vi "PAM Parse Other Data.vi"(1 "Header":string) -> (15 "Synchronization":T1, 16 "Magnetometer":T2, 17 "Acceleromter":T2)   [LabVIEW 2020]
panel:
  out "Sync Status":string
  out "System Time Status":string
  out "error out":errorcluster
  in  "error in (no error)":errorcluster
  out "Sync Offset":u32
  out "PPS Count":u32
  out "PPS Count":string
  out "Sync Offset":string
  out "Instrument Time":string
  out "Instrument Date":string
  out "Mag Z":i16
  out "Mag Y":i16
  out "Mag X":i16
  out "Accel Z":i16
  out "Accel Y":i16
  out "Accel X":i16
  out "Heading":string
  out "Battery":string
  out "Time":string
  out "Trigger Status":string
  out "Temp, Humidity":string
  out "Other Data Header":string
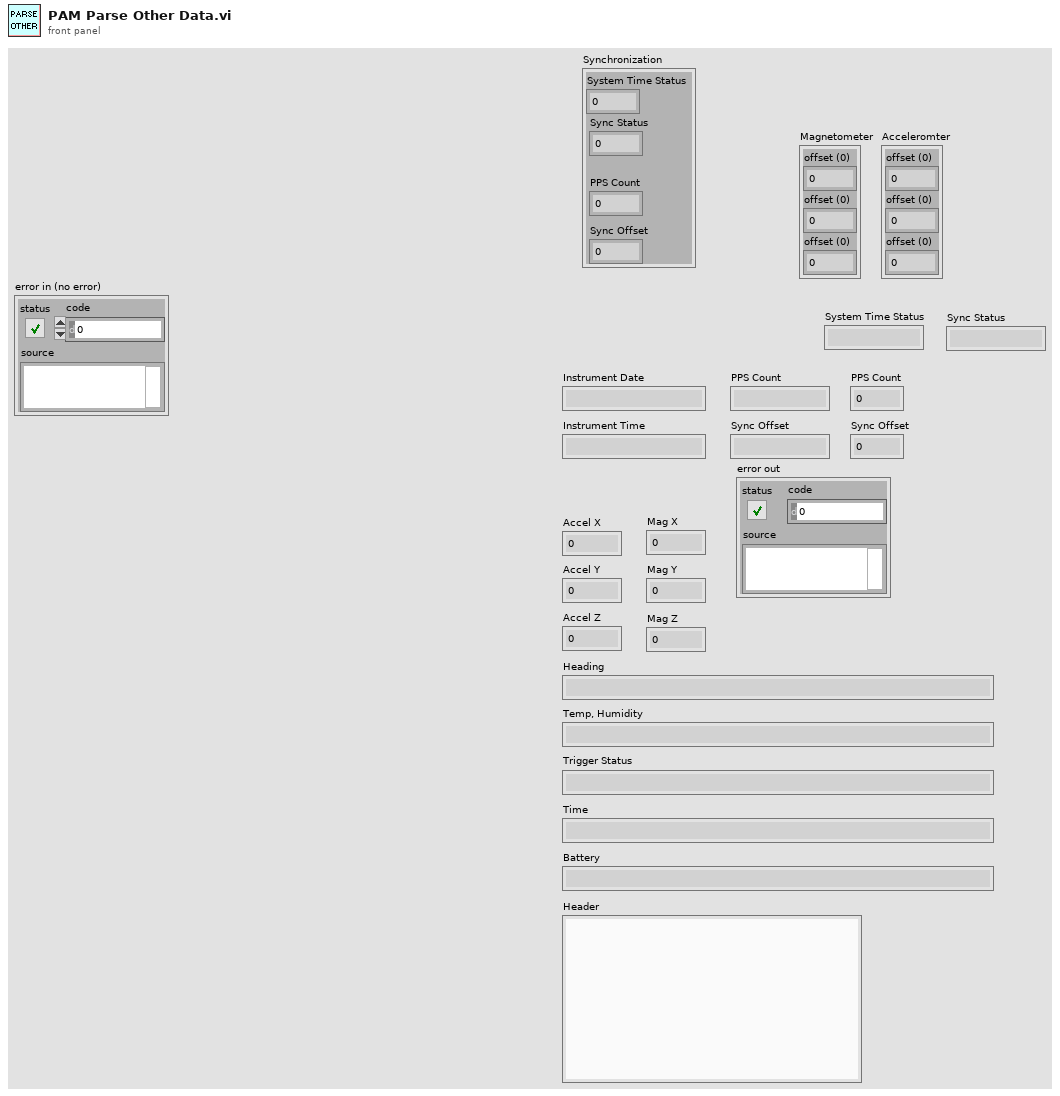
[diagram p1: front panel]
types:
  T1 = cluster{"System Time Status":u8, "Sync Status":u8, "PPS Count":u32, "Sync Offset":u32}
  T2 = cluster{"offset (0)":i16, "offset (0)":i16, "offset (0)":i16}
  T3 = enum16{"big-endian, network order", "native, host order", "little-endian"}
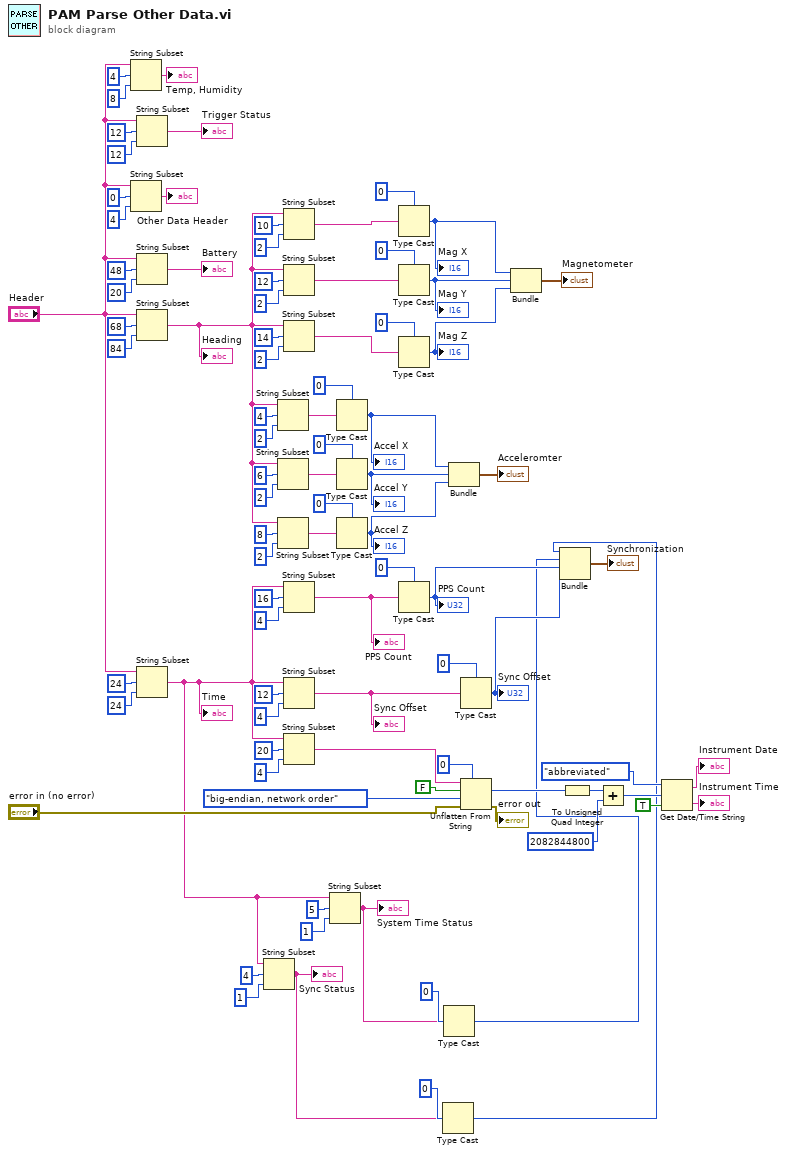
[diagram p0: block diagram]
diagram:
  n1 = String Subset(string="Header", offset (0)=4, length (rest)=8 ("length (rest)")) -> (substring=→"Temp, Humidity":string)
  n2 = String Subset(string="Header", offset (0)=0, length (rest)=4 ("length (rest)")) -> (substring=→"Other Data Header":string)
  n3 = String Subset(string="Header", offset (0)=12, length (rest)=12 ("offset (0)")) -> (substring=→"Trigger Status":string)
  n4 = String Subset(string="Header", offset (0)=48, length (rest)=20 ("offset (0)")) -> (substring=→"Battery":string)
  n5 = String Subset(string="Header", offset (0)=68, length (rest)=84 ("offset (0)")) -> (substring=w45:string)
  "Heading" <- w45
  n6 = String Subset(string="Header", offset (0)=24, length (rest)=24 ("offset (0)")) -> (substring=w8:string)
  "Time" <- w8
  n7 = String Subset(string=w8, offset (0)=4, length (rest)=1 ("offset (0)")) -> (substring=w4:string)
  "Sync Status" <- w4
  n8 = String Subset(string=w45, offset (0)=4, length (rest)=2 ("offset (0)")) -> (substring=w66:string)
  n9 = String Subset(string=w45, offset (0)=6, length (rest)=2 ("offset (0)")) -> (substring=w62:string)
  n10 = String Subset(string=w45, offset (0)=8, length (rest)=2 ("offset (0)")) -> (substring=w58:string)
  n11 = String Subset(string=w45, offset (0)=10, length (rest)=2 ("offset (0)")) -> (substring=w54:string)
  n12 = String Subset(string=w45, offset (0)=12, length (rest)=2 ("offset (0)")) -> (substring=w50:string)
  n13 = String Subset(string=w45, offset (0)=14, length (rest)=2 ("offset (0)")) -> (substring=w46:string)
  n14 = String Subset(string=w8, offset (0)=16, length (rest)=4 ("offset (0)")) -> (substring=w28:string)
  "PPS Count" <- w28
  n15 = String Subset(string=w8, offset (0)=12, length (rest)=4 ("offset (0)")) -> (substring=w25:string)
  "Sync Offset" <- w25
  n16 = String Subset(string=w8, offset (0)=20, length (rest)=4 ("offset (0)")) -> (substring=w37:string)
  n17 = String Subset(string=w8, offset (0)=5, length (rest)=1 ("offset (0)")) -> (substring=w6:string)
  "System Time Status" <- w6
  n18 = Type Cast(type=i16 0 ("offset (0)"), x=w66) -> (*(type *) &x=w18:i16)
  "Accel X" <- w18
  n19 = Type Cast(type=i16 0 ("offset (0)"), x=w62) -> (*(type *) &x=w15:i16)
  "Accel Y" <- w15
  n20 = Type Cast(type=i16 0 ("offset (0)"), x=w58) -> (*(type *) &x=w14:i16)
  "Accel Z" <- w14
  n21 = Type Cast(type=i16 0 ("offset (0)"), x=w54) -> (*(type *) &x=w20:i16)
  "Mag X" <- w20
  n22 = Type Cast(type=i16 0 ("offset (0)"), x=w50) -> (*(type *) &x=w19:i16)
  "Mag Y" <- w19
  n23 = Type Cast(type=i16 0 ("offset (0)"), x=w46) -> (*(type *) &x=w16:i16)
  "Mag Z" <- w16
  n24 = Type Cast(type=u32 0, x=w28) -> (*(type *) &x=w22:u32)
  "PPS Count" <- w22
  n25 = Type Cast(type=u8 0, x=w4) -> (*(type *) &x=w3:u8)
  n26 = Type Cast(type=u8 0, x=w6) -> (*(type *) &x=w2:u8)
  n27 = Bundle("offset (0)"=w18, "offset (0)"=w15, "offset (0)"=w14) -> (→"Acceleromter":T2)  [unwired: 1 in]
  n28 = Type Cast(type=u32 0, x=w25) -> (*(type *) &x=w21:u32)
  "Sync Offset" <- w21
  n29 = Unflatten From String(type=u32 0, binary string=w37, data includes array or string size? (T)=FALSE, byte order (0:big-endian, network order)=T3."big-endian, network order", error in (no error)="error in (no error)") -> (value=w33:u32, error out=→"error out":errorcluster)  [unwired: 1 out]
  n30 = Bundle("offset (0)"=w20, "offset (0)"=w19, "offset (0)"=w16) -> (→"Magnetometer":T2)  [unwired: 1 in]
  n31 = Bundle(w3, w2, w22, w21) -> (→"Synchronization":cluster{u8, u8, u32, u32})  [unwired: 1 in]
  n32 = To Unsigned Quad Integer(1:w33) -> (0:w38:u64)
  n33 = Add(x=w38, y=u64 2082844800) -> (x+y=w41:u64)
  n34 = Get Date/Time String(date format (0)=enum16{"short", "long", "abbreviated"}."abbreviated", seconds (now)=w41, want seconds? (F)=TRUE) -> (date string=→"Instrument Date":string, time string=→"Instrument Time":string)
